vi "n set wobbel.vi"(8 "error in (no error)":errorcluster, 9 "frequency":dbl, 10 "amplitude":u16, 11 "n":u16) -> (0 "error out":errorcluster)   [LabVIEW 2015, in "SCANalone4x64.lvlib"]
doc: "__declspec(dllimport) void __stdcall n_set_wobbel(unsigned short n, unsigned short amplitude, double frequency);"
uses:
  <userlib>/SCANalone4x64/SCANalone4x64.lvlib
  <userlib>/SCANalone4x64/SCANalone4x64.dll
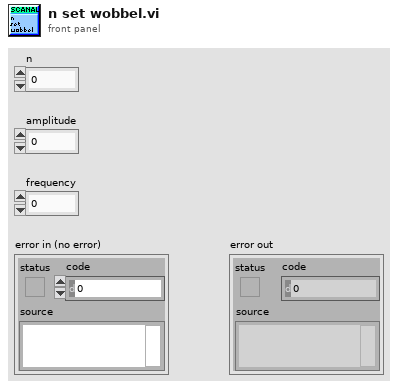
[diagram p1: front panel]
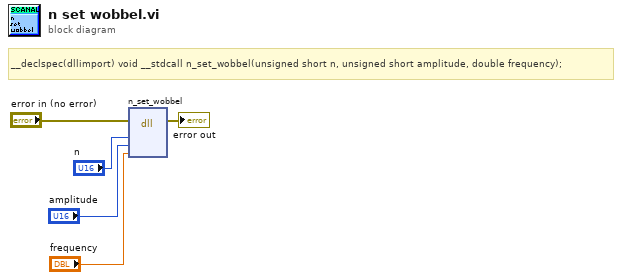
[diagram p0: block diagram]
diagram:
  # "__declspec(dllimport) void __stdcall n_set_wobbel(unsigned short n, unsigned short amplitude, double frequency);"
  n1 = dll-call lib="C:/Program Files/National Instruments/LabVIEW 2015/user.lib/SCANalone4x64/SCANalone4x64.*" fn="n_set_wobbel"(error in="error in (no error)", "n"="n", "amplitude"="amplitude", "frequency"="frequency") -> (error out=→"error out":errorcluster)  [unwired: 6 in, 1 out]
